vi "Generic.vi"(8 "error in":errorcluster, 11 "reference":refnum<vi>) -> (0 "error out":errorcluster, 3 "object out":refnum<class "Generic.lvclass">)   [LabVIEW 2014, in "Raspberry Pi Compatible Compiler for LabVIEW.lvlib" / "Generic.lvclass"]
uses:
  Generic.lvclass
  GObject/GObject.lvclass
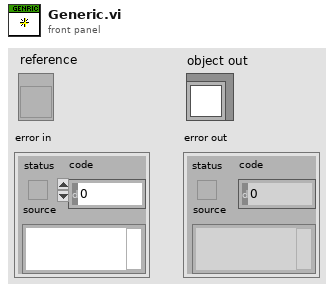
[diagram p1: front panel]
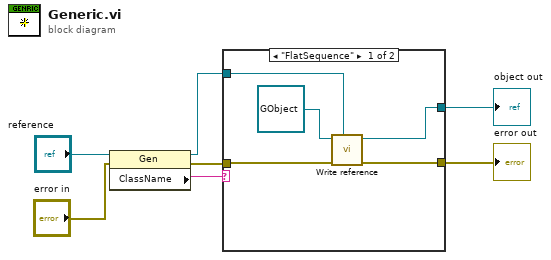
[diagram p0: block diagram]
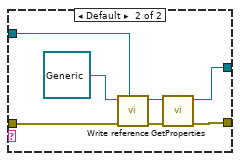
[diagram p2: hidden frame]
diagram:
  n1 = property class="Gen"(reference="reference", error in="error in") -> (reference out=w4:refnum<vi>, error out=w3:errorcluster, "ClassName"=w5:string)
  n2 = case shown="\"FlatSequence\"" w5 {
    tunnel: w4 -> [w10 w17]
    tunnel: w3 -> [w11 w18]
    tunnel: [w9 w14] -> w1
    tunnel: [w8 w13] -> w2
    frame "FlatSequence" {
      n3 = call-dynamic "Write reference.vi"("reference"=w10, "error in"=w11, "GObject in"=refnum<class "GObject.lvclass"> refnum) -> ("error out"=w9:errorcluster, "GObject out"=w8:refnum<class "GObject.lvclass">)  [unwired: 5 in]
    }
    frame Default {
      n4 = call-dynamic "Write reference.vi"("reference"=w17, "error in"=w18, "GObject in"=refnum<class "Generic.lvclass"> refnum) -> ("error out"=w15:errorcluster, "GObject out"=w16:refnum<class "Generic.lvclass">)  [unwired: 5 in]
      n5 = call-dynamic "GetProperties.vi"("error in"=w15, "Generic in"=w16) -> ("error out"=w14:errorcluster, "Generic out"=w13:refnum<class "Generic.lvclass">)  [unwired: 8 in]
    }
  }
  "error out" <- w1
  "object out" <- w2
